vi "read_cred_xml_no_details.vi"(5 "error in":errorcluster, 8 "XML File Path":path=path "C:/Users/Fielding/Documents/GitHub/Acquire_MAP_copy/ignore/creds.xml") -> (0 "error out":errorcluster, 1 "storage":T4, 2 "slack":T4, 3 "database_inf":T1)   [LabVIEW 2020]
uses:
  Type defs/cred_ctrl.ctl
  Type defs/data_cred.ctl
  Type defs/cred_ip_info.ctl
  DataBase/MYsql/lv_mysql_connector_v1_lv8/typedefs/mysql_authentication.ctl
  <vilib>/NI/GXML/_subVIs/GXML SearchParser/Search Parser.vi
  <vilib>/NI/GXML/GXML.lvlib
panel:
  out "database":T4
  out "XML String Out":string
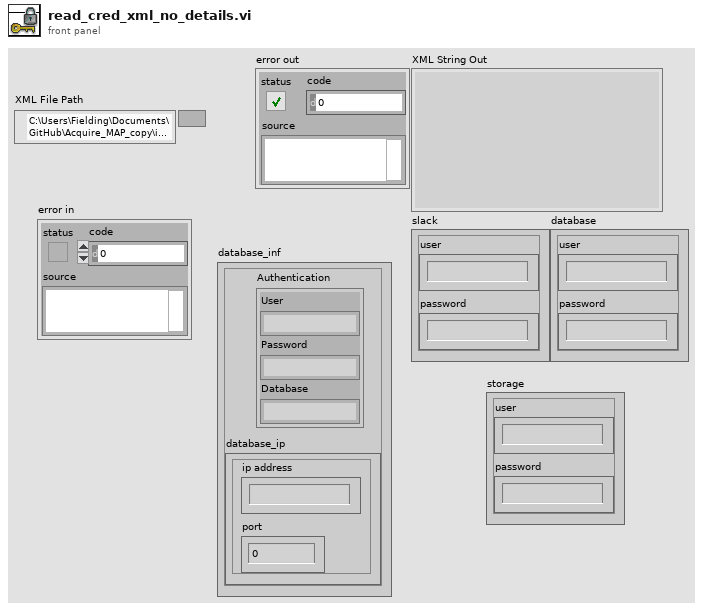
[diagram p1: front panel]
types:
  T1 = typedef "data_cred.ctl" = cluster{"database_ip":T2, "Authentication":T3}
  T2 = typedef "cred_ip_info.ctl" = cluster{"ip address":string, "port":dbl}
  T3 = typedef "mysql_authentication.ctl" = cluster{"User":string, "Password":string, "Database":string}
  T4 = typedef "cred_ctrl.ctl" = cluster{"user":string, "password":string}
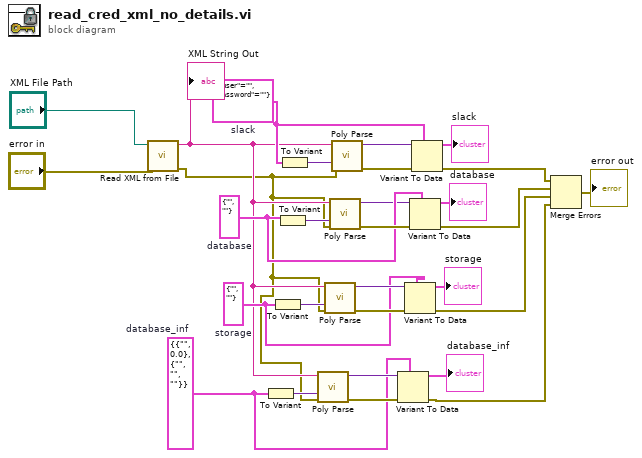
[diagram p0: block diagram]
diagram:
  w2 = T1 {"database_ip"={"ip address"="", "port"=0.0}, "Authentication"={"User"="", "Password"="", "Database"=""}}  # database_inf
  w13 = T4 {"user"="", "password"=""}  # storage
  w20 = T4 {"user"="", "password"=""}  # database
  w24 = T4 {"user"="", "password"=""}  # slack
  n1 = call <vilib>:"Read XML from File.vi"("error in"="error in", "XML File Path"="XML File Path") -> ("error out"=w6:errorcluster, "XML String Out"=w7:string)  [unwired: 8 in]
  "XML String Out" <- w7
  n2 = To Variant(anything=w2) -> (Variant=w8:variant)
  n3 = To Variant(anything=w13) -> (Variant=w15:variant)
  n4 = To Variant(anything=w20) -> (Variant=w21:variant)
  n5 = To Variant(anything=w24) -> (Variant=w27:variant)
  n6 = call-poly <vilib>:"Poly Parse.vi"("error in"=w6, "TypeDesc"=w8, "XML String In"=w7) -> ("error out"=w4:errorcluster, "Parsed Data"=w5:variant)  [unwired: 7 in]
  n7 = call-poly <vilib>:"Poly Parse.vi"("error in"=w6, "TypeDesc"=w15, "XML String In"=w7) -> ("error out"=w14:errorcluster, "Parsed Data"=w16:variant)  [unwired: 7 in]
  n8 = call-poly <vilib>:"Poly Parse.vi"("error in"=w6, "TypeDesc"=w21, "XML String In"=w7) -> ("error out"=w22:errorcluster, "Parsed Data"=w19:variant)  [unwired: 7 in]
  n9 = call-poly <vilib>:"Poly Parse.vi"("error in"=w6, "TypeDesc"=w27, "XML String In"=w7) -> ("error out"=w25:errorcluster, "Parsed Data"=w26:variant)  [unwired: 7 in]
  n10 = Variant To Data(error in=w4, type=w2, Variant=w5) -> (data=→"database_inf":T1, error out=w3:errorcluster)
  n11 = Variant To Data(error in=w14, type=w13, Variant=w16) -> (data=→"storage":T4, error out=w10:errorcluster)
  n12 = Variant To Data(error in=w22, type=w20, Variant=w19) -> (data=→"database":T4, error out=w11:errorcluster)
  n13 = Variant To Data(error in=w25, type=w24, Variant=w26) -> (data=→"slack":T4, error out=w12:errorcluster)
  n14 = Merge Errors(w12, w11, w10, w3) -> (→"error out":errorcluster)
